vi "setpoint(SubVI).vi"(0 "Filed 2":dbl=300.0, 1 "Field":dbl=300.0, 2 "类型":enum16{"temp", "field", "position"}(ring), 3 "Rate/speed":dbl=10.0, 4 "Mode":i32(ring) items=["Persistent", "Driven"], 6 "data":refnum<queue>, 7 "Delay":dbl, 9 "steps number":i32, 11 "Approach":i32(ring) items=["FastSettle", "NoOvershoot"], 15 "config":refnum<queue>) -> (8 "错误输出":errorcluster)   [LabVIEW 2019, in "SubVI.lvlib"]
uses:
  SubVI.lvlib
  config.ctl
  Instrument.ctl
  lib/QDInstrument.dll
  <vilib>/NI/Modbus Library/API/Master/Modbus Master.lvclass
panel:
  out "数组":dbl[](array[numeric])
  # "(真是通道1，假是通道2)"
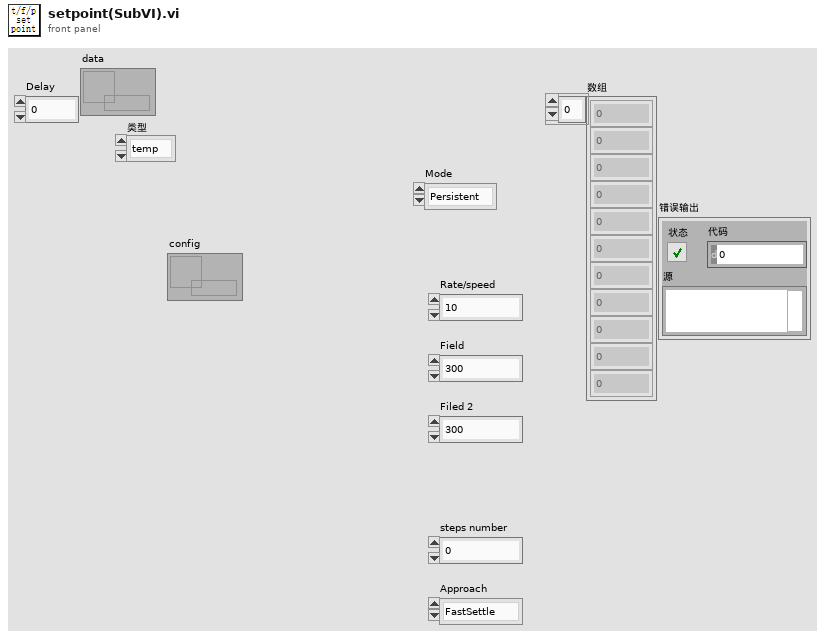
[diagram p1: front panel]
types:
  T1 = typedef "config.ctl" = cluster{"initialize":string, "6221":cluster{"6221 Resource":refnum<visa-resource-name>, "Delta status":bool}, "7001":cluster{"Ch":bool}, "SR830+6221":cluster{"source":u16, "阻抗":dbl, "量程入 4":i32, "量程入 3":i32, "量程入 2":i32, "量程入 1":i32, "电流":dbl, "SR830 2":bool, "SR830 3":bool, "SR830 4":bool, "SR830 1":bool, "VISA 1":refnum<visa-resource-name>, "VISA 2":refnum<visa-resource-name>, "VISA 3":refnum<visa-resource-name>, "VISA 4":refnum<visa-resource-name>, "量程":enum16{"量程每次测量会判定", "量程不变为设定值"}}, "2400":cluster{"2400":bool, "VISA":refnum<visa-resource-name>}, "ch":cluster{"ch str":string, "ch1":bool, "ch2":bool, "布尔":bool}, "error":bool, "数据文件路径":path, "log":cluster{"log路径":path, "log interval":dbl}, "Instrument":T2}
  T2 = typedef "Instrument.ctl" = cluster{"335 Resource":refnum<visa-resource-name>, "Input (0:A)":u16, "Instrument Type":i32, "quantum design":refnum<k24>, "Heater Output (1:1)":u16, "335state":refnum<vi>, "semaphore":T3, "TCP master instance":refnum<class "Modbus Master.lvclass">}
  T3 = typedef "Semaphore RefNum" = refnum<k1>
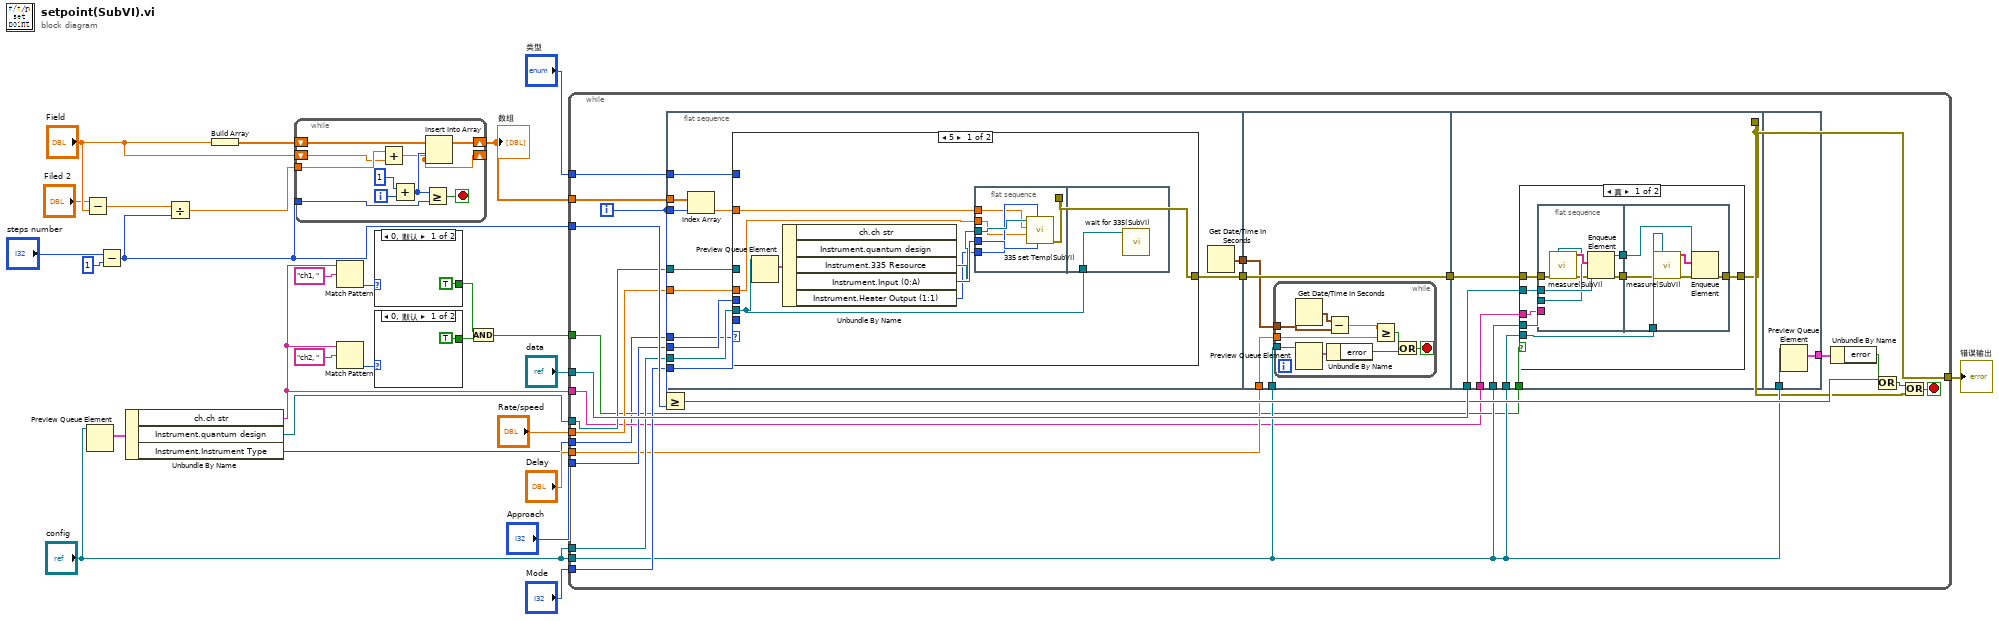
[diagram p0: block diagram]
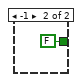
[diagram p2: hidden frame]
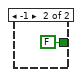
[diagram p3: hidden frame]
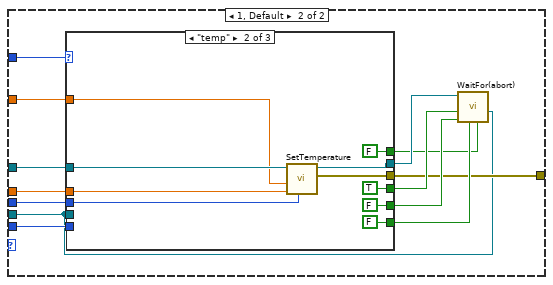
[diagram p4: hidden frame]
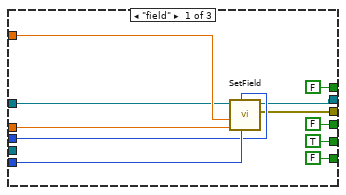
[diagram p5: hidden frame]
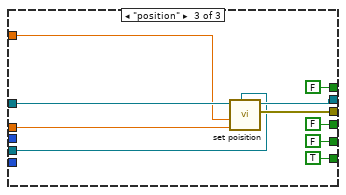
[diagram p6: hidden frame]
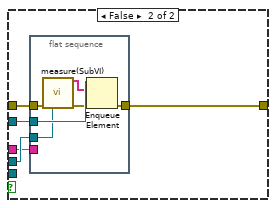
[diagram p7: hidden frame]
diagram:
  n1 = Subtract(x="Filed 2", y="Field") -> (x-y=w25:dbl)
  n2 = Preview Queue Element(queue="config") -> (element=w4:T1)  [unwired: 2 in, 3 out]
  n3 = Subtract(x="steps number", y=1) -> (x-y=w16:i32)
  n4 = Unbundle By Name(w4) -> ("ch.ch str"=w3:string, "Instrument.quantum design"=w2:refnum<k24>, "Instrument.Instrument Type"=w1:i32)
  n5 = Divide(x=w25, y=w16) -> (x/y=w27:dbl)
  n6 = Build Array("Field") -> (w26:dbl[])
  n7 = while {
    shift-right: [w38] -> w20
    shift-left: w26 -> [w37]
    tunnel: w27 -> [w32]
    tunnel: w16 -> [w31]
    shift-right: [w30] -> _
    shift-left: "Field" -> [w29]
    i -> [w36]
    stop <- w33 stop-if-true
    n8 = Add(x=w32, y=w29) -> (x+y=w30:dbl)
    n9 = Add(x=1, y=w36) -> (x+y=w34:i32)
    n10 = Greater Or Equal?(x=w34, y=w31) -> (x >= y?=w33:bool)
    n11 = Insert Into Array(array=w37, index=w34, new element=w30) -> (w38:dbl[])
  }
  "数组" <- w20
  n12 = Match Pattern(string=w3, regular expression="ch1, " ("正则表达式")) -> (offset past match=w10:i32)  [unwired: 1 in, 3 out]
  n13 = Match Pattern(string=w3, regular expression="ch2, " ("正则表达式")) -> (offset past match=w9:i32)  [unwired: 1 in, 3 out]
  n14 = case shown="0, 默认" w10 {
    tunnel: [TRUE FALSE] -> w8
    frame 0, Default {
    }
    frame -1 {
    }
  }
  n15 = case shown="0, 默认" w9 {
    tunnel: [TRUE FALSE] -> w7
    frame 0, Default {
    }
    frame -1 {
    }
  }
  n16 = And(x=w8, y=w7) -> (x .and. y?=w6:bool)
  n17 = while {
    tunnel: w16 -> [w64]
    tunnel: "data" -> [w66]
    tunnel: "config" -> [w50]
    tunnel: "Mode" -> [w62]
    tunnel: "Approach" -> [w61]
    tunnel: "Rate/speed" -> [w60]
    tunnel: w2 -> [w59]
    tunnel: w20 -> [w58]
    tunnel: "config" -> [w57]
    tunnel: [w49] -> w19
    tunnel: "Delay" -> [w51]
    tunnel: "类型" -> [w46]
    tunnel: w6 -> [w45]
    tunnel: w3 -> [w44]
    tunnel: w1 -> [w43]
    i -> [w63]
    stop <- w55 stop-if-true
    n18 = Greater Or Equal?(x=w63, y=w64) -> (x >= y?=w65:bool)
    n19 = flat-sequence {
      tunnel: w63 -> [w73]
      tunnel: w62 -> [w77]
      tunnel: w61 -> [w76]
      tunnel: w60 -> [w75]
      tunnel: w59 -> [w72]
      tunnel: w58 -> [w74]
      tunnel: w57 -> [w68]
      tunnel: [w71] -> w54
      tunnel: [w70] -> w52
      tunnel: w46 -> [w69]
      tunnel: w43 -> [w67]
      tunnel: w54 -> [w141]
      tunnel: [w141] -> w53
      tunnel: w52 -> [w140]
      tunnel: w51 -> [w138]
      tunnel: w50 -> [w139]
      tunnel: w50 -> [w154]
      tunnel: [w153] -> w49
      tunnel: w53 -> [w156]
      tunnel: w50 -> [w155]
      tunnel: w66 -> [w157]
      tunnel: w45 -> [w152]
      tunnel: w44 -> [w151]
      tunnel: w50 -> [w191]
      tunnel: [w190] -> w48
      frame #0 {
        n20 = Index Array(array=w74, index=w73) -> (element=w78:dbl)
        n21 = case shown="5" w67 {
          tunnel: w78 -> [w82 w106]
          tunnel: w77 -> [_ w105]
          tunnel: w76 -> [_ w104]
          tunnel: w75 -> [w81 w103]
          tunnel: w72 -> [_ w102]
          tunnel: [w80 w96] -> w71
          tunnel: w69 -> [_ w95]
          tunnel: w68 -> [w79 w94]
          frame 5 {
            n22 = Preview Queue Element(queue=w79) -> (element=w86:T1)  [unwired: 2 in, 3 out]
            n23 = Unbundle By Name(w86) -> ("Instrument.335 Resource"=w85:refnum<visa-resource-name>, "Instrument.Input (0:A)"=w84:u16, "Instrument.Heater Output (1:1)"=w83:u16)  [unwired: 2 out]
            n24 = flat-sequence {
              tunnel: w85 -> [w92]
              tunnel: w84 -> [w91]
              tunnel: w83 -> [w90]
              tunnel: w82 -> [w89]
              tunnel: w81 -> [w88]
              tunnel: [w87] -> w80
              tunnel: w79 -> [w93]
              frame #0 {
                n25 = call "335 set Temp(SubVI).vi"("Input (0:A)"=w91, "Output (1:1)"=w90, "Rate"=w88, "Temperature"=w89, "VISA Refnum in"=w92) -> ("error out"=w87:errorcluster)  [unwired: 5 in, 1 out]
              }
              frame #1 {
                n26 = call "wait for 335(SubVI).vi"("队列输出"=w93) -> ()  [unwired: 11 in]
              }
            }
          }
          frame 1, Default {
            n27 = case shown="\"temp\"" w95 {
              tunnel: w106 -> [w117 w122 w130]
              tunnel: w105 -> [w116 _ _]
              tunnel: w104 -> [w115 w120 _]
              tunnel: w103 -> [w114 w121 w129]
              tunnel: w102 -> [w113 w123 w133]
              tunnel: [w112 w119 w132] -> w101
              tunnel: [FALSE ("Wait For Temperature") TRUE ("Wait For Temperature") FALSE ("Wait For Temperature")] -> w100
              tunnel: [TRUE ("Wait For Field") FALSE ("Wait For Field") FALSE ("Wait For Field")] -> w99
              tunnel: [FALSE ("Wait For Position") FALSE ("Wait For Position") TRUE ("Wait For Position")] -> w98
              tunnel: [FALSE ("Wait For Chamber") FALSE ("Wait For Chamber") FALSE ("Wait For Chamber")] -> w97
              tunnel: [w107 w118 w131] -> w96
              tunnel: w94 -> [_ _ w128]
              frame "field" {
                n28 = call "SetField.vi"("Mode"=w116, "Approach"=w115, "Rate"=w114, "Field"=w117, "Instrument Ref In"=w113) -> ("error out"=w107:errorcluster, "Instrument Ref Out"=w112:refnum<k24>)  [unwired: 2 in, 1 out]
              }
              frame "temp" {
                n29 = call "SetTemperature.vi"("Approach"=w120, "Rate"=w121, "Temperature"=w122, "Instrument Ref In"=w123) -> ("error out"=w118:errorcluster, "Instrument Ref Out"=w119:refnum<k24>)  [unwired: 3 in, 1 out]
              }
              frame "position" {
                n30 = call "set poisition.vi"("config"=w128, "Slow down code\ndefault = 0"=w129, "Position (deg)"=w130, "Instrument Ref In"=w133) -> ("error out"=w131:errorcluster, "Instrument Ref Out"=w132:refnum<k24>)  [unwired: 4 in]
              }
            }
            n31 = call "WaitFor(abort).vi"("config"=w94, "Wait For Chamber"=w97, "Wait For Position"=w98, "Wait For Field"=w99, "Wait For Temperature"=w100, "Instrument Ref In"=w101) -> ()  [unwired: 4 in, 2 out]
          }
        }
        n32 = Get Date/Time In Seconds() -> (seconds since 1Jan1904=w70:timestamp)
      }
      frame #1 {
        n33 = while {
          tunnel: w140 -> [w149]
          tunnel: w138 -> [w147]
          tunnel: w139 -> [w145]
          stop <- w143 stop-if-true
          n34 = Get Date/Time In Seconds() -> (seconds since 1Jan1904=w150:timestamp)
          n35 = Preview Queue Element(queue=w145) -> (element=w144:T1)  [unwired: 2 in, 3 out]
          n36 = Subtract(x=w150, y=w149) -> (x-y=w148:dbl)
          n37 = Unbundle By Name(w144) -> ("error"=w142:bool)
          n38 = Greater Or Equal?(x=w148, y=w147) -> (x >= y?=w146:bool)
          n39 = Or(x=w146, y=w142) -> (x .or. y?=w143:bool)
        }
      }
      frame #2 {
        n40 = case shown="真" w152 {
          tunnel: w157 -> [w163 w183]
          tunnel: w156 -> [w162 w182]
          tunnel: w155 -> [w161 w181]
          tunnel: w154 -> [w160 _]
          tunnel: [w159 w180] -> w153
          tunnel: w151 -> [w158 w179]
          frame True {
            n41 = flat-sequence {
              tunnel: w163 -> [w170]
              tunnel: w162 -> [w168]
              tunnel: w161 -> [w167]
              tunnel: [w172] -> w165
              tunnel: [w171] -> w164
              tunnel: w158 -> [_]
              tunnel: w165 -> [w176]
              tunnel: w164 -> [w177]
              tunnel: w160 -> [w178]
              tunnel: [w173] -> w159
              frame #0 {
                n42 = call "measure(SubVI).vi"("config"=w167, "error in (no error)"=w168) -> ("data"=w169:string[], "error out"=w166:errorcluster)  [unwired: 12 in]
                n43 = Enqueue Element(queue=w170, element=w169, error in (no error)=w166) -> (queue out=w172:refnum<queue>, error out=w171:errorcluster)  [unwired: 1 in, 1 out]
              }
              frame #1 {
                n44 = call "measure(SubVI).vi"("config"=w178, "error in (no error)"=w177) -> ("data"=w175:string[], "error out"=w174:errorcluster)  [unwired: 12 in]
                n45 = Enqueue Element(queue=w176, element=w175, error in (no error)=w174) -> (error out=w173:errorcluster)  [unwired: 1 in, 2 out]
              }
            }
          }
          frame False {
            n46 = flat-sequence {
              tunnel: [w189] -> w180
              tunnel: w179 -> [_]
              tunnel: w181 -> [w185]
              tunnel: w182 -> [w186]
              tunnel: w183 -> [w188]
              frame #0 {
                n47 = call "measure(SubVI).vi"("config"=w185, "error in (no error)"=w186) -> ("data"=w187:string[], "error out"=w184:errorcluster)  [unwired: 12 in]
                n48 = Enqueue Element(queue=w188, element=w187, error in (no error)=w184) -> (error out=w189:errorcluster)  [unwired: 1 in, 2 out]
              }
            }
          }
        }
      }
      frame #3 {
        n49 = Preview Queue Element(queue=w191) -> (element=w190:T1)  [unwired: 2 in, 3 out]
      }
    }
    n50 = Unbundle By Name(w48) -> ("error"=w47:bool)
    n51 = Or(x=w65, y=w47) -> (x .or. y?=w56:bool)
    n52 = Or(x=w56, y=w49) -> (x .or. y?=w55:bool)
  }
  "错误输出" <- w19
